vi "StringChannelSelector.vi"(7 "reference 2":refnum<vi>, 8 "error in (no error)":errorcluster, 11 "input string":string="1") -> (0 "error out":errorcluster, 3 "Channel Selection out":string)   [LabVIEW 2011]
uses:
  LVComboBoxStrsAndValuesArrayTypeDef.ctl
panel:
  out "Strings And Values []":T1
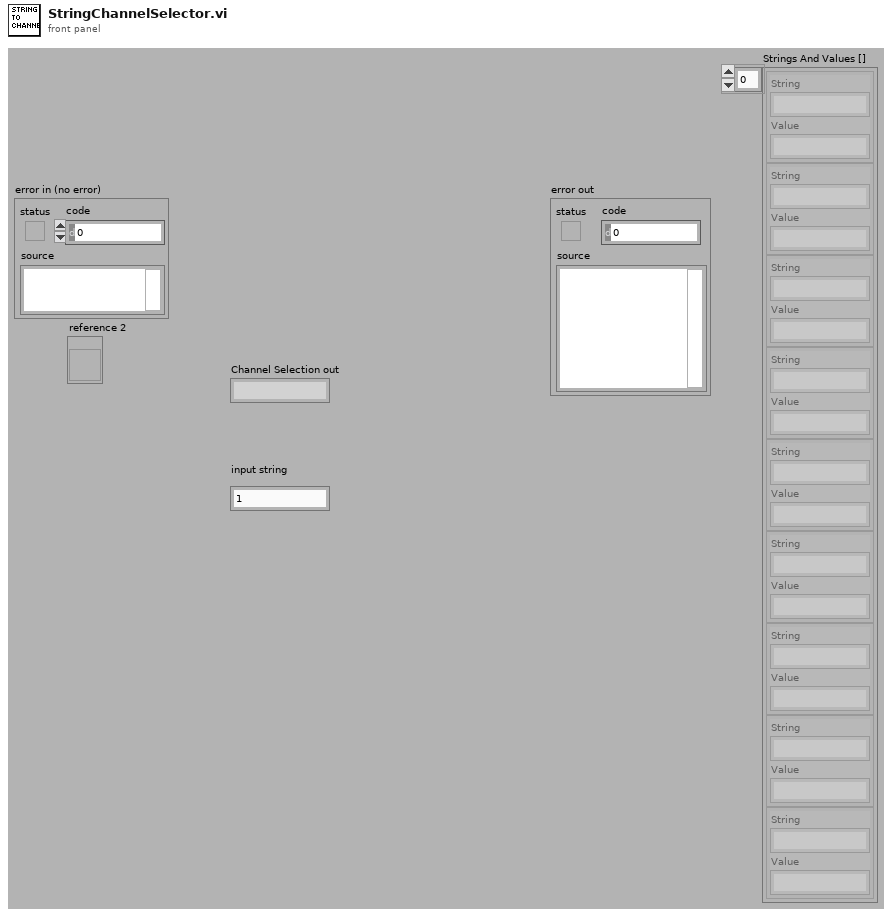
[diagram p1: front panel]
types:
  T1 = typedef "LVComboBoxStrsAndValuesArrayTypeDef.ctl" = cluster{"String":string, "Value":string}[]
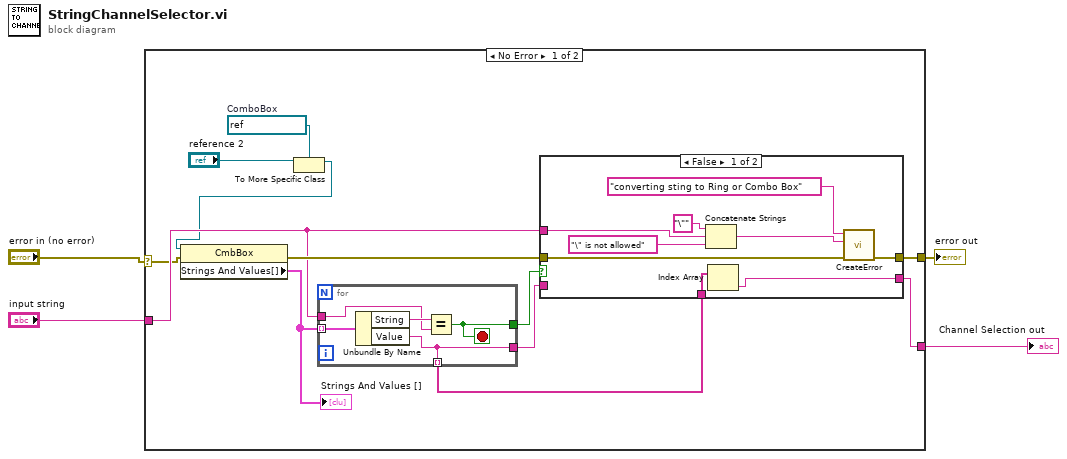
[diagram p0: block diagram]
diagram:
  n1 = case shown="No Error" "error in (no error)" {
    selector: "error in (no error)" -> [w11 w33]
    tunnel: [w6 w34] -> w4
    tunnel: "input string" -> [w13 w34]
    tunnel: [w12 w33] -> w2
    frame No Error {
      w9 = refnum<vi> refnum  # ComboBox
      n2 = To More Specific Class(target class=w9, reference="reference 2") -> (specific class reference=w8:refnum<vi>)  [unwired: 1 in, 1 out]
      n3 = property class="CmbBox"(reference=w8, error in=w11) -> (error out=w14:errorcluster, "Strings And Values[]"=w16:T1)  [unwired: 1 out]
      "Strings And Values []" <- w16
      n4 = for {
        tunnel: w16 -> [w32] mode=indexing
        tunnel: w13 -> [w30]
        tunnel: [w28] -> w7
        tunnel: [w29] -> w15
        tunnel: [w28] -> w5 mode=indexing
        stop <- w29 stop-if-true
        n5 = Unbundle By Name(w32) -> ("String"=w31:string, "Value"=w28:string)
        n6 = Equal?(x=w31, y=w30) -> (x = y?=w29:bool)
      }
      n7 = case shown="False" w15 {
        tunnel: w14 -> [w25 w27]
        tunnel: [w24 w27] -> w12
        tunnel: w13 -> [w22 _]
        tunnel: w7 -> [_ w26]
        tunnel: [w17 w26] -> w6
        tunnel: w5 -> [w18 _]
        frame False {
          n8 = Concatenate Strings("\"" ("string"), w22, "\" is not allowed" ("string")) -> (w19:string)
          n9 = Index Array(array=w18) -> (element=w17:string)  [unwired: 1 in]
          n10 = call "CreateError.vi"("user error in"=w25, "error message (\"\")"=w19, "command"="converting sting to Ring or Combo Box") -> ("user error  out"=w24:errorcluster)  [unwired: 8 in]
        }
        frame True {
        }
      }
    }
    frame Error {
    }
  }
  "Channel Selection out" <- w4
  "error out" <- w2
